vi "UPD Generate and Map Last Update Tag.vi"(8 "error in (no error)":errorcluster, 11 "node References":T1) -> (0 "error out":errorcluster, 3 "node References out":T1)   [LabVIEW 2015, in "E2E Tag Exchange editor node.lvclass"]
uses:
  E2E Tag Exchange editor node.lvclass
  object references.ctl
  <vilib>/NI/DCAF/Tag Editor Core/Configuration Editor/Classes/Engine Parent/Engine Parent Editor Node.lvclass
  <vilib>/NI/Module Execution Interface/Engine Configuration/engine configuration.lvclass
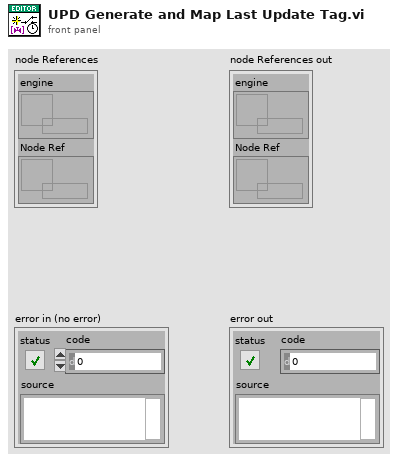
[diagram p1: front panel]
types:
  T1 = typedef "E2E Tag Exchange editor node.lvclass/object references.ctl" = cluster{"engine":refnum<data-value>, "Node Ref":refnum<data-value>}
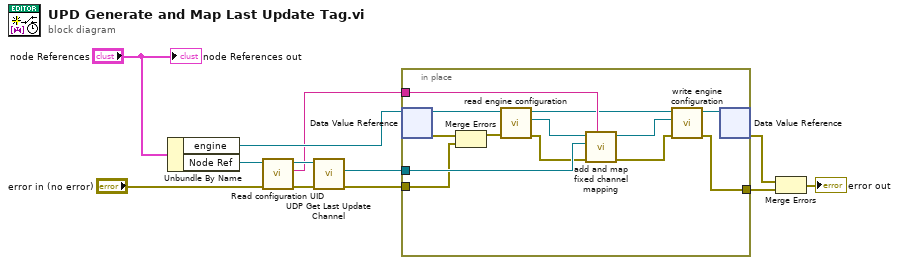
[diagram p0: block diagram]
diagram:
  n1 = Unbundle By Name("node References") -> ("engine"=w10:refnum<data-value>, "Node Ref"=w9:refnum<data-value>)
  n2 = call "Read configuration UID.vi"("error in (no error)"="error in (no error)", "E2E editor node in"=w9) -> ("error out"=w7:errorcluster, "Module UID"=w6:string, "E2E editor node out"=w8:refnum<data-value>)  [unwired: 7 in]
  n3 = call "UDP Get Last Update Channel.vi"("error in (no error)"=w7, "E2E editor node in"=w8) -> ("error out"=w5:errorcluster, "channel out"=w11:refnum<class "TBM channel.lvclass">)  [unwired: 7 in, 1 out]
  n4 = in-place {
    in-place-border: w11 -> [w25]
    in-place-border: w6 -> [w23]
    in-place-border: w5 -> [w18]
    in-place-border: [w15] -> w3
    n5 = in-place-dvr #1(w10) -> (w24:refnum<class "Engine Parent Editor Node.lvclass">, w17:errorcluster)
    n6 = Merge Errors(w17, w18) -> (w16:errorcluster)
    n7 = call <vilib>:"read engine configuration.vi"("error in"=w16, "Engine Parent Editor Node in"=w24) -> ("error out"=w13:errorcluster, "engine configuration"=w14:refnum<class "engine configuration.lvclass">, "Engine Parent Editor Node out"=w22:refnum<class "Engine Parent Editor Node.lvclass">)  [unwired: 7 in]
    n8 = call <vilib>:"add and map fixed channel mapping.vi"("module instance"=w23, "error in"=w13, "fixed channel"=w25, "engine configuration in"=w14) -> ("error out"=w20:errorcluster, "engine configuration out"=w19:refnum<class "engine configuration.lvclass">)  [unwired: 6 in]
    n9 = call <vilib>:"write engine configuration.vi"("error in"=w20, "engine configuration"=w19, "Engine Parent Editor Node in"=w22) -> ("error out"=w15:errorcluster, "Engine Parent Editor Node out"=w21:refnum<class "Engine Parent Editor Node.lvclass">)  [unwired: 7 in]
    n10 = in-place-dvr #1(w21) -> (w2:errorcluster)  [unwired: 1 out]
  }
  n11 = Merge Errors(w2, w3) -> (→"error out":errorcluster)
  "node References out" <- "node References"
